vi "Merge Err.vi"(8 "error in (no error)":errorcluster, 11 "return type":i32) -> (0 "error out":errorcluster)   [LabVIEW 2015, in "mcp2210.lvlib"]
uses:
  <userlib>/mcp2210/mcp2210.lvlib
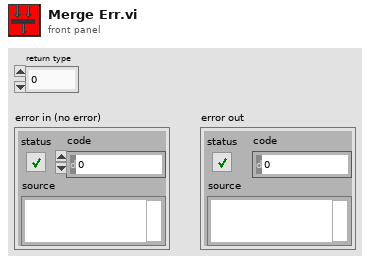
[diagram p1: front panel]
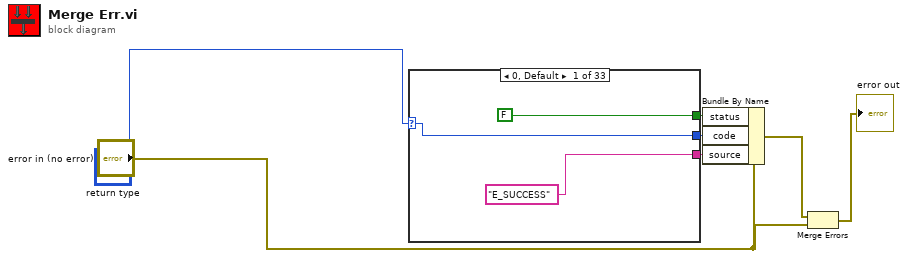
[diagram p0: block diagram]
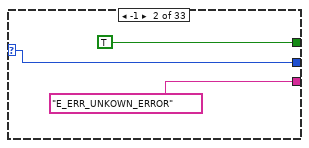
[diagram p2: hidden frame]
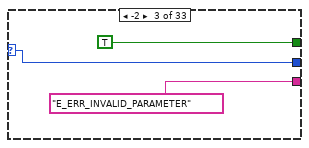
[diagram p3: hidden frame]
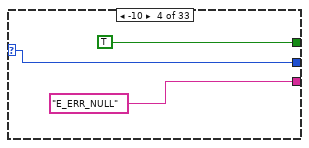
[diagram p4: hidden frame]
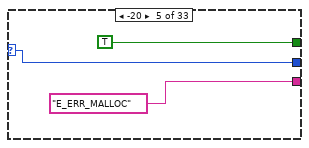
[diagram p5: hidden frame]
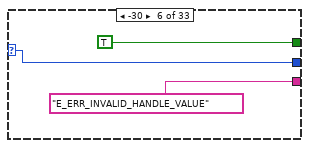
[diagram p6: hidden frame]
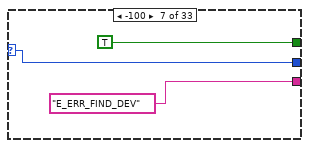
[diagram p7: hidden frame]
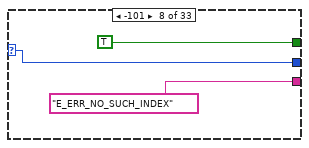
[diagram p8: hidden frame]
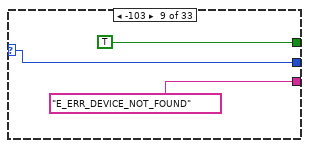
[diagram p9: hidden frame]
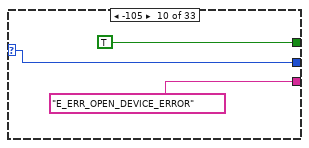
[diagram p10: hidden frame]
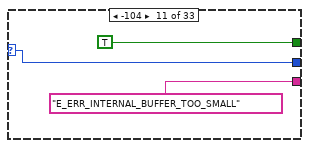
[diagram p11: hidden frame]
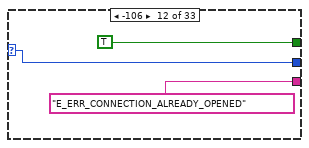
[diagram p12: hidden frame]
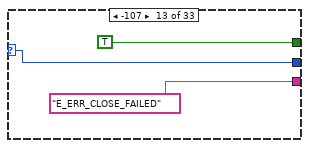
[diagram p13: hidden frame]
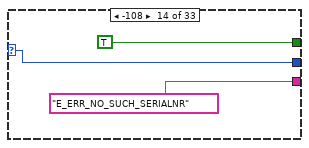
[diagram p14: hidden frame]
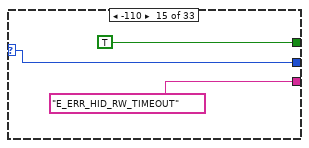
[diagram p15: hidden frame]
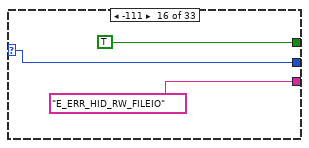
[diagram p16: hidden frame]
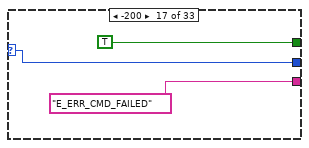
[diagram p17: hidden frame]
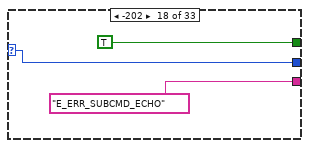
[diagram p18: hidden frame]
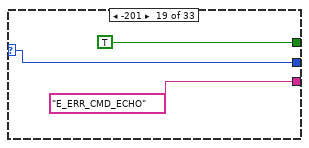
[diagram p19: hidden frame]
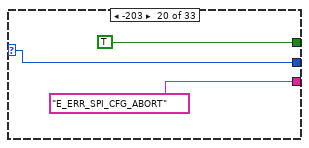
[diagram p20: hidden frame]
diagram:
  n1 = case shown="0, Default" "return type" {
    selector: "return type" -> [w9 w12 w15 w18 w21 w24 w27 w30 w33 w36 w39 w42 w45 w48 w51 w54 w57 w60 w63 w66 w69 w72 w75 w78 w81 w84 w87 w90 w93 w96 w99 w102 w105]
    tunnel: [FALSE TRUE TRUE TRUE TRUE TRUE TRUE TRUE TRUE TRUE TRUE TRUE TRUE TRUE TRUE TRUE TRUE TRUE TRUE TRUE TRUE TRUE TRUE TRUE TRUE TRUE TRUE TRUE TRUE TRUE TRUE TRUE TRUE] -> w2
    tunnel: [w9 w12 w15 w18 w21 w24 w27 w30 w33 w36 w39 w42 w45 w48 w51 w54 w57 w60 w63 w66 w69 w72 w75 w78 w81 w84 w87 w90 w93 w96 w99 w102 w105] -> w3
    tunnel: ["E_SUCCESS" "E_ERR_UNKOWN_ERROR" "E_ERR_INVALID_PARAMETER" "E_ERR_NULL" "E_ERR_MALLOC" "E_ERR_INVALID_HANDLE_VALUE" "E_ERR_FIND_DEV" "E_ERR_NO_SUCH_INDEX" "E_ERR_DEVICE_NOT_FOUND" "E_ERR_OPEN_DEVICE_ERROR" "E_ERR_INTERNAL_BUFFER_TOO_SMALL" "E_ERR_CONNECTION_ALREADY_OPENED" "E_ERR_CLOSE_FAILED" "E_ERR_NO_SUCH_SERIALNR" "E_ERR_HID_RW_TIMEOUT" "E_ERR_HID_RW_FILEIO" "E_ERR_CMD_FAILED" "E_ERR_SUBCMD_ECHO" "E_ERR_CMD_ECHO" "E_ERR_SPI_CFG_ABORT" "E_ERR_SPI_EXTERN_MASTER" "E_ERR_SPI_TIMEOUT" "E_ERR_SPI_RX_INCOMPLETE" "E_ERR_SPI_XFER_ONGOING" "E_ERR_BLOCKED_ACCESS" "E_ERR_EEPROM_WRITE_FAIL" "E_ERR_NVRAM_LOCKED" "E_ERR_WRONG_PASSWD" "E_ERR_ACCESS_DENIED" "E_ERR_NVRAM_PROTECTED" "E_ERR_PASSWD_CHANGE" "E_ERR_STRING_DESCRIPTOR" "E_ERR_STRING_TOO_LARGE"] -> w4
    frame 0, Default {
    }
    frame -1 {
    }
    frame -2 {
    }
    frame -10 {
    }
    frame -20 {
    }
    frame -30 {
    }
    frame -100 {
    }
    frame -101 {
    }
    frame -103 {
    }
    frame -105 {
    }
    frame -104 {
    }
    frame -106 {
    }
    frame -107 {
    }
    frame -108 {
    }
    frame -110 {
    }
    frame -111 {
    }
    frame -200 {
    }
    frame -202 {
    }
    frame -201 {
    }
    frame -203 {
    }
    frame -204 {
    }
    frame -205 {
    }
    frame -206 {
    }
    frame -207 {
    }
    frame -300 {
    }
    frame -301 {
    }
    frame -350 {
    }
    frame -351 {
    }
    frame -352 {
    }
    frame -353 {
    }
    frame -354 {
    }
    frame -400 {
    }
    frame -401 {
    }
  }
  n2 = Bundle By Name(cluster="error in (no error)", "status"=w2, "code"=w3, "source"=w4) -> (w5:errorcluster)
  n3 = Merge Errors(w5, "error in (no error)") -> (→"error out":errorcluster)
